vi "Solution part 2a.vi"(11 "data?":bool) -> ()   [LabVIEW 2020]
panel:
  out "sum of memory":u64
  out "mask for setting":u64 format="%.0b"
  out "mask len ok?":bool
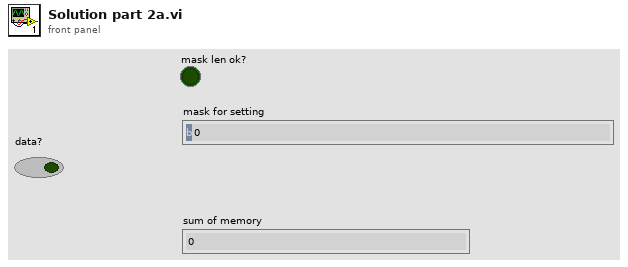
[diagram p1: front panel]
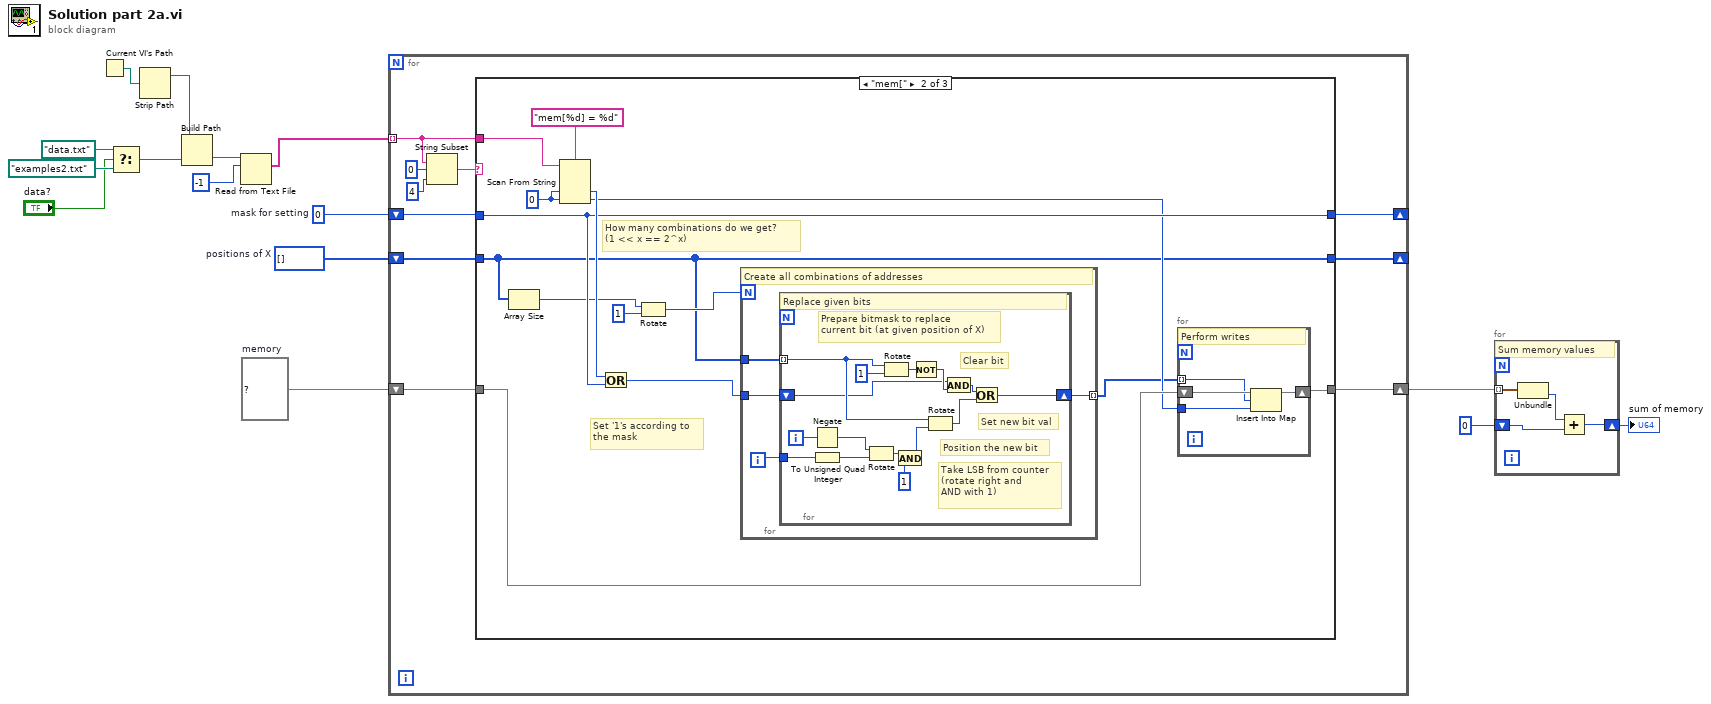
[diagram p0: block diagram]
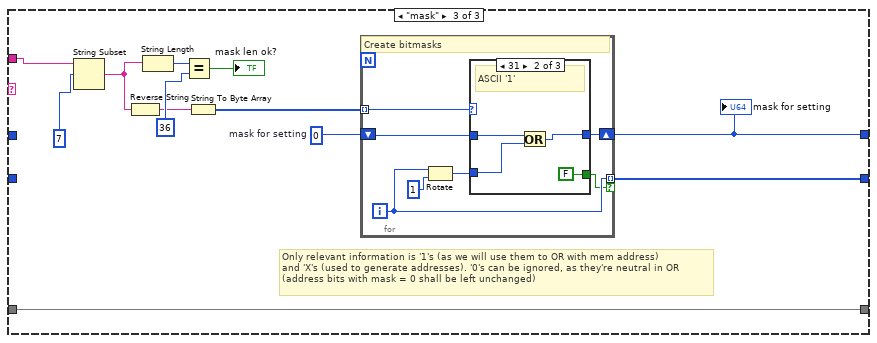
[diagram p3: hidden frame]
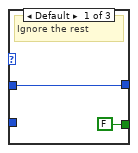
[diagram p4: hidden frame]
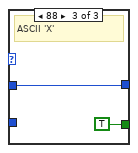
[diagram p5: hidden frame]
diagram:
  w1 = i32[] []  # positions of X
  w4 = u64 0  # mask for setting
  w3 = map{u64, u64} {}  # memory
  n1 = Current VI's Path() -> (path=w12:path)
  n2 = Select(t=path "data.txt", s="data?", f=path "examples2.txt") -> (s? t:f=w13:path)
  n3 = Strip Path(path=w12) -> (stripped path=w11:path)  [unwired: 1 out]
  n4 = Build Path(base path=w11, name or relative path=w13) -> (appended path=w10:path)
  n5 = Read from Text File(file (use dialog)=w10, count=-1) -> (text=w5:string[])  [unwired: 2 in, 3 out]
  n6 = for {
    tunnel: w5 -> [w18] mode=indexing
    shift-right: [w21] -> _
    shift-left: w4 -> [w22]
    shift-right: [w19] -> w2
    shift-left: w3 -> [w20]
    shift-right: [w16] -> _
    shift-left: w1 -> [w17]
    n7 = String Subset(string=w18, offset (0)=0, length (rest)=4 ("length (rest)")) -> (substring=w23:string)
    n8 = case shown="\"mem[\"" w23 {
      tunnel: w22 -> [w28 w38 _]
      tunnel: [w28 w38 w72] -> w21
      tunnel: w20 -> [w27 w36 w71]
      tunnel: [w27 w37 w71] -> w19
      tunnel: w18 -> [_ w40 w70]
      tunnel: w17 -> [w26 w31 _]
      tunnel: [w26 w31 w66] -> w16
      frame Default {
      }
      frame "mem[" {
        w41 = u64 0 ("default value 2")
        # "How many combinations do we get?\n(1 << x == 2^x)"
        # "Set '1's according to \nthe mask"
        n9 = Array Size(array=w31) -> (size(s)=w33:i32)
        n10 = Scan From String(format string="mem[%d] = %d", input string=w40, default 1=w41, default 2=w41) -> (output 1=w39:u64, output 2=w35:u64)  [unwired: 2 in, 3 out]
        n11 = Or(x=w39, y=w38) -> (x .or. y?=w30:u64)
        n12 = Rotate(1:u32 1 ("x"), 2:w33) -> (0:w32:u32)
        n13 = for {
          N: w32 -> [_]
          tunnel: w31 -> [w46]
          tunnel: w30 -> [w44]
          tunnel: [w43] -> w29 mode=indexing
          i -> [w45]
          # "Create all combinations of addresses"
          n14 = for {
            tunnel: w45 -> [w60]
            tunnel: w46 -> [w57] mode=indexing
            shift-right: [w51] -> w43
            shift-left: w44 -> [w54]
            i -> [w49]
            # "Position the new bit"
            # "Set new bit val"
            # "Clear bit"
            # "Prepare bitmask to replace\ncurrent bit (at given position of X)"
            # "Take LSB from counter\n(rotate right and \nAND with 1)"
            # "Replace given bits"
            n15 = Negate(x=w49) -> (-x=w61:i32)
            n16 = To Unsigned Quad Integer(1:w60) -> (0:w50:u64)
            n17 = Rotate(1:w50, 2:w61) -> (0:w59:u64)
            n18 = Rotate(1:u64 1 ("x"), 2:w57) -> (0:w56:u64)
            n19 = And(x=w59, y=u64 1) -> (x .and. y?=w48:u64)
            n20 = Not(x=w56) -> (.not. x?=w55:u64)
            n21 = Rotate(1:w48, 2:w57) -> (0:w52:u64)
            n22 = And(x=w54, y=w55) -> (x .and. y?=w53:u64)
            n23 = Or(x=w53, y=w52) -> (x .or. y?=w51:u64)
          }
        }
        n24 = for {
          shift-right: [w65] -> w37
          shift-left: w36 -> [w64]
          tunnel: w35 -> [w63]
          tunnel: w29 -> [w62] mode=indexing
          # "Perform writes"
          n25 = Insert Into Map(map in=w64, key=w62, value=w63) -> (map out=w65:map{u64, u64})  [unwired: 2 out]
        }
      }
      frame "mask" {
        w69 = u64 0  # mask for setting
        # "Only relevant information is '1's (as we will use them to OR with mem address)\nand 'X's (used to generate addresses). '0's can be ignored, as they're neutral in OR \n(address bits with mask = 0 shall be left unchanged)"
        n26 = String Subset(string=w70, offset (0)=7) -> (substring=w68:string)  [unwired: 1 in]
        n27 = Reverse String(1:w68) -> (0:w67:string)
        n28 = String Length(string=w68) -> (length=w76:i32)
        n29 = Equal?(x=w76, y=36) -> (x = y?=→"mask len ok?":bool)
        n30 = String To Byte Array(string=w67) -> (unsigned byte array=w75:u8[])
        n31 = for {
          tunnel: w75 -> [w84] mode=indexing
          shift-right: [w80] -> w72
          shift-left: w69 -> [w83]
          tunnel: [w79] -> w66 mode=indexing if=w78
          i -> [w79]
          # "Create bitmasks"
          n32 = Rotate(1:u64 1 ("x"), 2:w79) -> (0:w81:u64)
          n33 = case shown="31" w84 {
            tunnel: w83 -> [w86 w90 w92]
            tunnel: w81 -> [_ w89 _]
            tunnel: [w86 w88 w92] -> w80
            tunnel: [FALSE FALSE TRUE] -> w78
            frame Default {
              # "Ignore the rest"
            }
            frame 49 {
              # "ASCII '1'"
              n34 = Or(x=w90, y=w89) -> (x .or. y?=w88:u64)
            }
            frame 88 {
              # "ASCII 'X'"
            }
          }
        }
        "mask for setting" <- w72
      }
    }
  }
  n35 = for {
    shift-right: [w96] -> w6
    shift-left: u64 0 ("default value 2") -> [w94]
    tunnel: w2 -> [w93] mode=indexing
    # "Sum memory values"
    n36 = Unbundle(w93) -> (w95:u64)  [unwired: 1 out]
    n37 = Add(x=w95, y=w94) -> (x+y=w96:u64)
  }
  "sum of memory" <- w6
